vi "Write Poll Rate.vi"(8 "error in (no error)":errorcluster, 10 "Poll Rate":i64, 11 "Level Controller in":refnum<class "Timed Loop Actor.lvclass">) -> (0 "error out":errorcluster, 3 "Level Controller out":refnum<class "Timed Loop Actor.lvclass">)   [LabVIEW 2025, in "Timed Loop Actor.lvlib" / "Timed Loop Actor.lvclass"]
doc: "Sets the time interval used for each iteration of the loop."
uses:
  Timed Loop Actor.lvclass
  Timed Loop Actor.lvclass/Timed Loop Actor.ctl
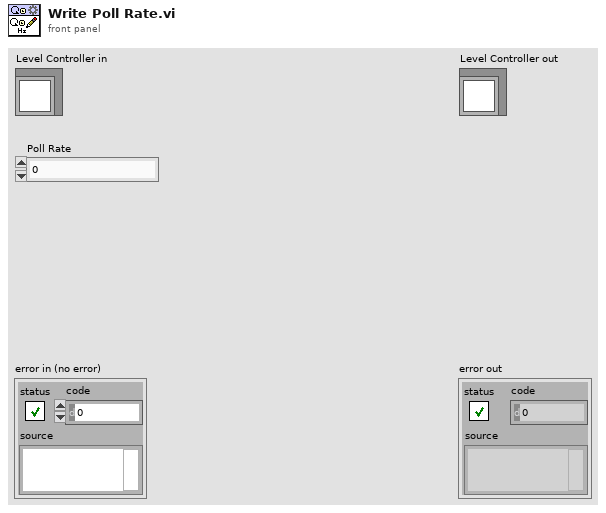
[diagram p1: front panel]
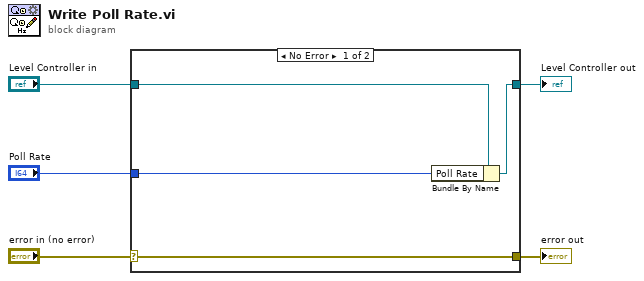
[diagram p0: block diagram]
diagram:
  n1 = case shown="No Error" "error in (no error)" {
    selector: "error in (no error)" -> [w9 w10]
    tunnel: [w9 w10] -> w4
    tunnel: [w7 w11] -> w2
    tunnel: "Level Controller in" -> [w8 w11]
    tunnel: "Poll Rate" -> [w6 _]
    frame No Error {
      n2 = Bundle By Name(cluster=w8, "Poll Rate"=w6) -> (w7:refnum<class "Timed Loop Actor.lvclass">)
    }
    frame Error {
    }
  }
  "error out" <- w4
  "Level Controller out" <- w2
